vi "ROI Description to ROI.vi"(8 "error in (no error)":errorcluster, 11 "ROI Description":string) -> (0 "error out":errorcluster, 3 "Current ROI Descriptor(s)":T3 {"Contours"."Type" items=["No Selection", "Point", "Line", "Rectangle", "Oval", "Polygon", "Freehand Region", "Annulus", "Unused2", "Unused3", "Broken Line", "Freehand Line", "Rotated Rectangle"]})   [LabVIEW 2021, in "Image.lvlib"]
uses:
  Image.lvlib
  Image ROI Type.ctl
  ROI Description Analysis Step.ctl
  <vilib>/regexp/Match Regular Expression.xnode
panel:
  in  "Contour":T1 {"Type" items=["No Selection", "Point", "Line", "Rectangle", "Oval", "Polygon", "Freehand Region", "Annulus", "Unused2", "Unused3", "Broken Line", "Freehand Line", "Rotated Rectangle"]}
  in  "ROI Type":T2
  out "ROI Name":string
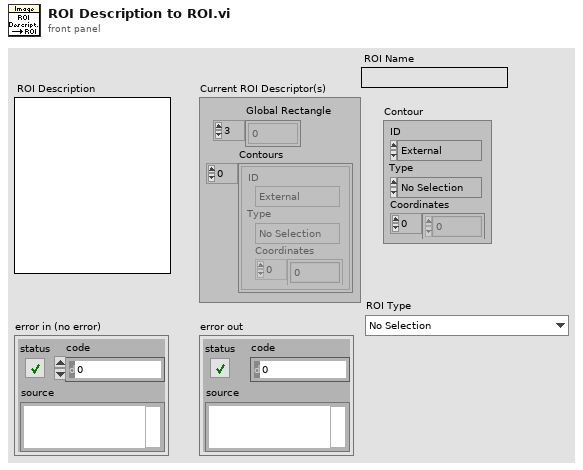
[diagram p1: front panel]
types:
  T1 = cluster{"ID":enum32{"External", "Internal"}, "Type":u32, "Coordinates":i32[]}
  T2 = typedef "Image.lvlib/Image ROI Type.ctl" = enum16{"No Selection", "Point", "Line", "Rectangle", "Oval", "Polygon", "Freehand Region", "Annulus", "Unused2", "Unused3", "Broken Line", "Freehand Line", "Rotated Rectangle"}
  T3 = typedef "ROI Descriptor" = cluster{"Global Rectangle":i32[], "Contours":cluster{"ID":enum32{"External", "Internal"}, "Type":u32, "Coordinates":i32[]}[]}
  T4 = typedef "Image.lvlib/ROI Description Analysis Step.ctl" = enum16{"ROI Name", "ROI Source", "Number of pixels", "Global Rectangle", "Number of Countours", "End"}
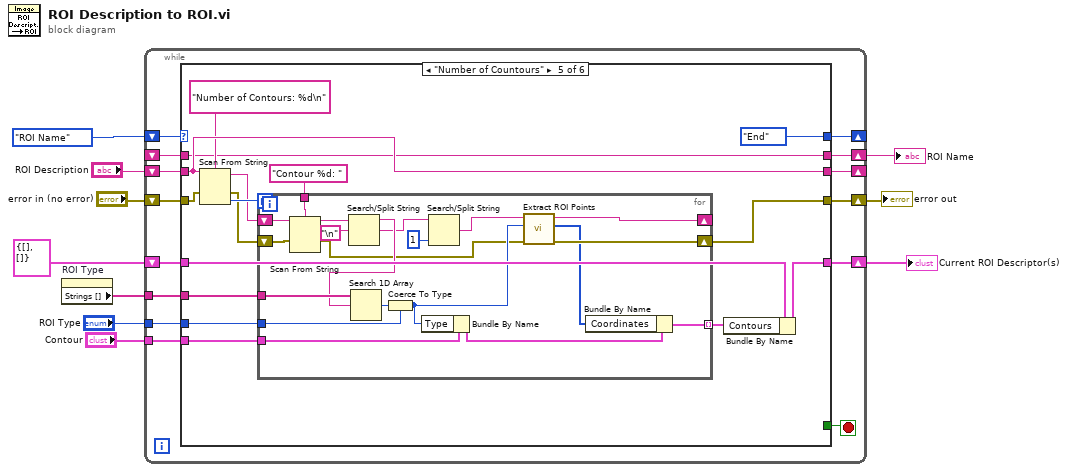
[diagram p0: block diagram]
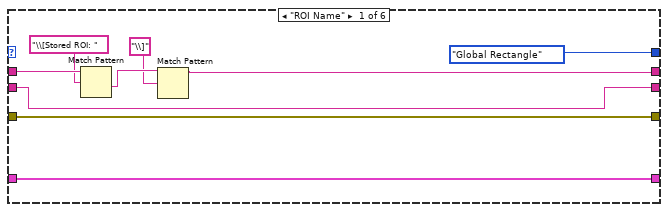
[diagram p2: hidden frame]
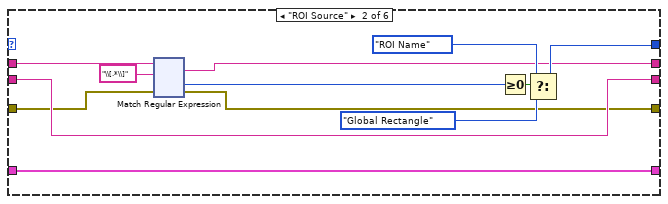
[diagram p3: hidden frame]
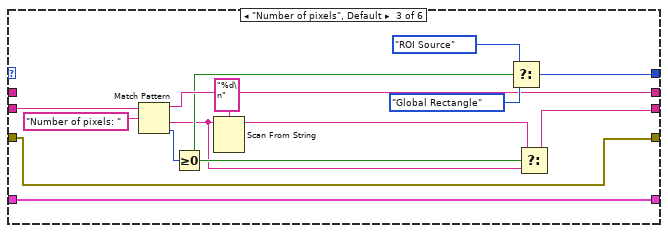
[diagram p4: hidden frame]
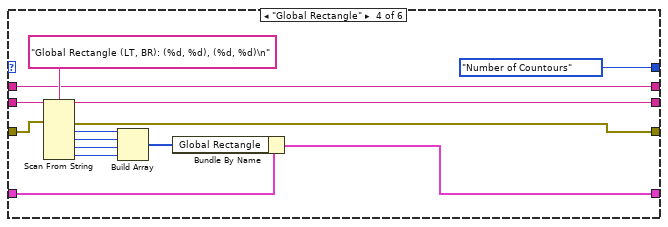
[diagram p5: hidden frame]
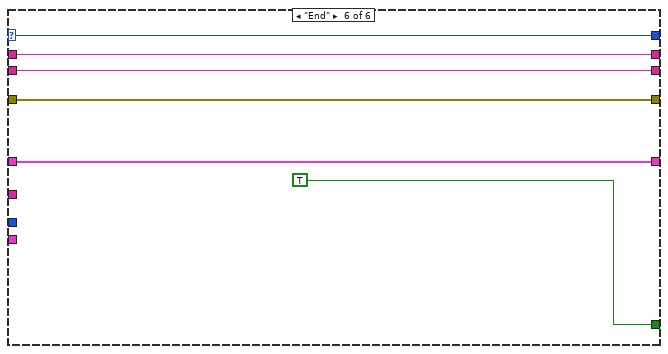
[diagram p6: hidden frame]
diagram:
  n1 = property on="ROI Type" class="Enum (strict)"() -> ("Strings []"=w4:string[])  [unwired: 2 in, 2 out]
  n2 = while {
    shift-right: [w19] -> _
    shift-left: "ROI Description" -> [w24]
    shift-right: [w22] -> _
    shift-left: ROI_Description_Analysis_Step."ROI Name" -> [w23]
    shift-right: [w21] -> w5
    shift-left: _ -> [w20]
    shift-right: [w17] -> w8
    shift-left: T3 {"Global Rectangle"=[], "Contours"=[]} ("Current ROI Descriptor(s)") -> [w18]
    shift-right: [w15] -> w6
    shift-left: "error in (no error)" -> [w16]
    tunnel: w4 -> [w13]
    tunnel: "Contour" -> [w12]
    tunnel: "ROI Type" -> [w11]
    stop <- w14 stop-if-true
    n3 = case shown="\"Number of Countours\"" w23 {
      selector: w23 -> [_ _ _ _ _ w230]
      tunnel: w24 -> [w32 w39 w176 w190 w206 w229]
      tunnel: [ROI_Description_Analysis_Step."Global Rectangle" w40 w171 ROI_Description_Analysis_Step."Number of Countours" ROI_Description_Analysis_Step."End" w230] -> w22
      tunnel: [w26 w35 w168 w188 w204 w232] -> w21
      tunnel: w20 -> [w30 w34 _ w188 w204 w232]
      tunnel: [w32 w39 w163 w177 w206 w229] -> w19
      tunnel: w18 -> [w31 w38 w170 w187 w202 w231]
      tunnel: [w31 w38 w170 w186 w193 w231] -> w17
      tunnel: w16 -> [w25 w37 w169 w179 w199 w228]
      tunnel: [w25 w36 w169 w178 w197 w228] -> w15
      tunnel: [_ _ _ _ _ TRUE] -> w14
      tunnel: w13 -> [_ _ _ _ w195 _]
      tunnel: w12 -> [_ _ _ _ w194 _]
      tunnel: w11 -> [_ _ _ _ w191 _]
      frame "ROI Name" {
        n4 = Match Pattern(string=w30, regular expression="\\[Stored ROI: " ("format string")) -> (after substring=w28:string)  [unwired: 1 in, 3 out]
        n5 = Match Pattern(string=w28, regular expression="\\]") -> (before substring=w26:string)  [unwired: 1 in, 3 out]
      }
      frame "ROI Source" {
        n6 = xnode "Match Regular Expression"("input string"=w34, "regular expression"="\\[.*\\]", "error in"=w37) -> ("whole match"=w35:string, "offset past match"=w44:i32, "error out"=w36:errorcluster)  [unwired: 3 in, 2 out]
        n7 = Greater Or Equal To 0?(x=w44) -> (x >= 0?=w43:bool)
        n8 = Select(t=ROI_Description_Analysis_Step."ROI Name", s=w43, f=ROI_Description_Analysis_Step."Global Rectangle") -> (s? t:f=w40:T4)
      }
      frame "Number of pixels", Default {
        n9 = Match Pattern(string=w176, regular expression="Number of pixels: ") -> (before substring=w168:string, after substring=w164:string, offset past match=w174:i32)  [unwired: 1 in, 1 out]
        n10 = Greater Or Equal To 0?(x=w174) -> (x >= 0?=w167:bool)
        n11 = Scan From String(format string="%d\n", input string=w164) -> (remaining string=w165:string)  [unwired: 4 in, 2 out]
        n12 = Select(t=ROI_Description_Analysis_Step."ROI Source", s=w167, f=ROI_Description_Analysis_Step."Global Rectangle") -> (s? t:f=w171:T4)
        n13 = Select(t=w165, s=w167, f=w164) -> (s? t:f=w163:string)
      }
      frame "Global Rectangle" {
        n14 = Scan From String(format string="Global Rectangle (LT, BR): (%d, %d), (%d, %d)\n" ("regular expression"), input string=w190, error in=w179) -> (remaining string=w177:string, error out=w178:errorcluster, output 1=w185:i32, output 2=w184:i32, output 3=w183:i32, output 4=w182:i32)  [unwired: 5 in, 1 out]
        n15 = Build Array(w185, w184, w183, w182) -> (w181:i32[])
        n16 = Bundle By Name(cluster=w187, "Global Rectangle"=w181) -> (w186:T3)
      }
      frame "Number of Countours" {
        n17 = Scan From String(format string="Number of Contours: %d\n" ("regular expression"), input string=w206, error in=w199) -> (remaining string=w196:string, error out=w198:errorcluster, output 1=w201:i32)  [unwired: 2 in, 1 out]
        n18 = for {
          N: w201 -> [_]
          shift-right: [w218] -> _
          shift-left: w196 -> [w226]
          tunnel: "Contour %d: " ("format string") -> [w225]
          shift-right: [w215] -> w197
          shift-left: w198 -> [w224]
          tunnel: w195 -> [w223]
          tunnel: w194 -> [w222]
          tunnel: [w216] -> w192 mode=indexing
          tunnel: w191 -> [w219]
          n19 = Scan From String(format string=w225, input string=w226, error in=w224) -> (remaining string=w214:string, error out=w208:errorcluster)  [unwired: 3 in, 1 out]
          n20 = Search/Split String(string=w214, search string/char (-)="\n") -> (substring before match=w213:string, match + rest of string=w211:string)  [unwired: 1 in, 1 out]
          n21 = Search 1D Array(1D array=w223, element=w213) -> (index of element=w221:i32)  [unwired: 1 in]
          n22 = Coerce To Type(0:w221, 1:w219) -> (2:w220:T2)
          n23 = Bundle By Name(cluster=w222, "Type"=w220) -> (w217:T1)
          n24 = Search/Split String(string=w211, offset (0)=1) -> (match + rest of string=w209:string)  [unwired: 1 in, 2 out]
          n25 = call "Extract ROI Points.vi"("error in (no error)"=w208, "ROI Type"=w220, "String in"=w209) -> ("error out"=w215:errorcluster, "Coordinates"=w207:i32[], "String out"=w218:string)  [unwired: 6 in]
          n26 = Bundle By Name(cluster=w217, "Coordinates"=w207) -> (w216:T1)
        }
        n27 = Bundle By Name(cluster=w202, "Contours"=w192) -> (w193:T3)
      }
      frame "End" {
      }
    }
  }
  "Current ROI Descriptor(s)" <- w8
  "error out" <- w6
  "ROI Name" <- w5
